vi "Array station.vi"() -> ()   [LabVIEW 2018]
panel:
  in  "Humidité":dbl[](array[numeric])
  in  "Pression":dbl[](array[numeric])
  in  "Température":dbl[](array[numeric])
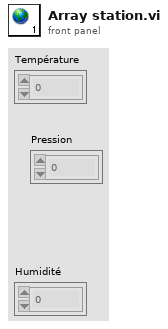
[diagram p1: front panel]
diagram:
